vi "chr63204A_Load_State_read.vi"(8 "error in (no error)":errorcluster, 11 "VISA resource name":refnum<visa-resource-name>) -> (0 "error out":errorcluster, 2 "LOAD_STATE":bool, 3 "VISA resource name out":refnum<visa-resource-name>)   [LabVIEW 2020]
doc: "Sets the voltage to be loaded on chroma 63204A"
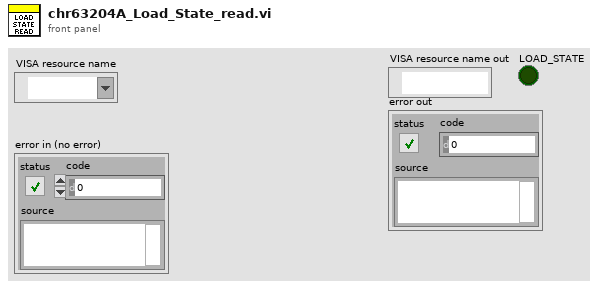
[diagram p1: front panel]
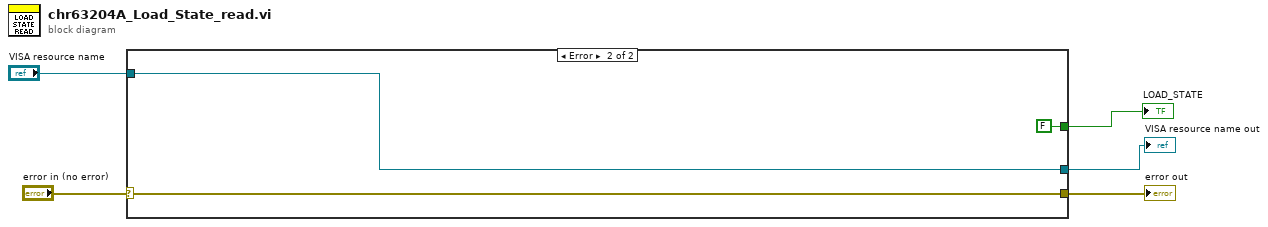
[diagram p0: block diagram]
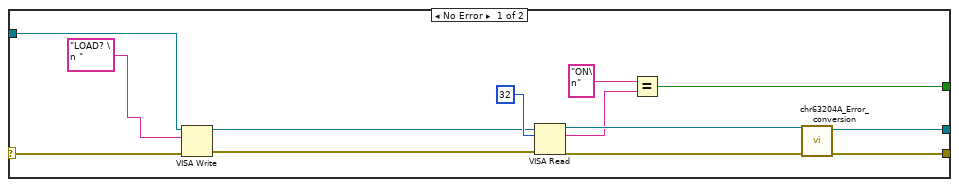
[diagram p2: hidden frame]
diagram:
  n1 = case shown="Error" "error in (no error)" {
    selector: "error in (no error)" -> [w17 w20]
    tunnel: "VISA resource name" -> [w18 w21]
    tunnel: [w16 w21] -> w3
    tunnel: [w15 w20] -> w2
    tunnel: [w6 FALSE] -> w1
    frame No Error {
      n2 = VISA Write(VISA resource name=w18, write buffer="LOAD? \n " ("string"), error in (no error)=w17) -> (VISA resource name out=w9:refnum<visa-resource-name>, error out=w10:errorcluster)  [unwired: 1 out]
      n3 = VISA Read(VISA resource name=w9, byte count=u32 32, error in (no error)=w10) -> (VISA resource name out=w12:refnum<visa-resource-name>, read buffer=w8:string, error out=w11:errorcluster)  [unwired: 1 out]
      n4 = Equal?(x="ON\n", y=w8) -> (x = y?=w6:bool)
      n5 = call "chr63204A_Error_conversion.vi"("error in (no error)"=w11, "VISA resource name"=w12) -> ("error out"=w15:errorcluster, "VISA resource name out"=w16:refnum<visa-resource-name>)  [unwired: 8 in]
    }
    frame Error {
    }
  }
  "VISA resource name out" <- w3
  "error out" <- w2
  "LOAD_STATE" <- w1
